vi "readTelemetryDynamicData.vi"(8 "error in (no error)":errorcluster, 10 "Parser":refnum<class "U8ArrayParserAutoIndexing.lvclass">, 11 "M1M3SAL in":refnum<class "M1M3SAL.lvclass">) -> (0 "error out":errorcluster, 2 "EventSummaryState":variant, 3 "M1M3SAL out":refnum<class "M1M3SAL.lvclass">)   [LabVIEW 2016, in "M1M3SupportCommunicator.lvlib" / "M1M3SAL.lvclass"]
uses:
  M1M3SAL.lvclass
  Common_RT_Utilities/U8ArrayParserAutoIndexing/U8ArrayParserAutoIndexing.lvclass
  DataTypes/Topics/TelemetryDynamicData.ctl
  DataTypes/Topics/Parts/Timestamp.ctl
  DataTypes/Topics/M1M3SupportTopics.lvlib
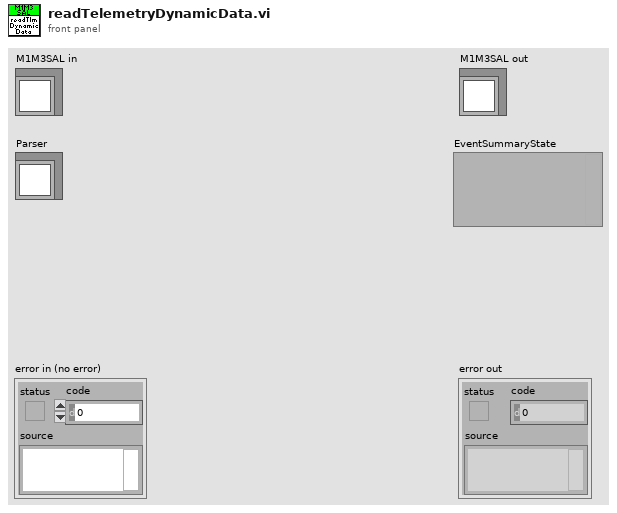
[diagram p1: front panel]
types:
  T1 = typedef "M1M3SupportTopics.lvlib/TelemetryDynamicData.ctl" = cluster{"Timestamp":T2, "AzimuthVelocity":dbl, "ElevationVelocity":dbl, "AzimuthAcceleration":dbl, "ElevationAcceleration":dbl}
  T2 = typedef "M1M3SupportTopics.lvlib/Timestamp.ctl" = dbl
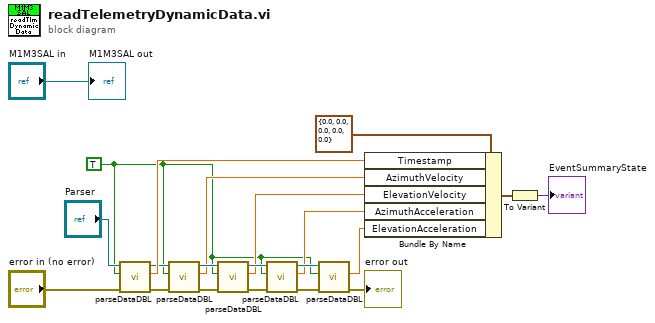
[diagram p0: block diagram]
diagram:
  w1 = TRUE ("OverrideSwapBytes")
  n1 = call "parseDataDBL.vi"("error in (no error)"="error in (no error)", "OverrideSwapBytes"=w1, "U8ArrayParserAutoIndexing in"="Parser") -> ("error out"=w9:errorcluster, "Data"=w16:dbl, "U8ArrayParserAutoIndexing out"=w11:refnum<class "U8ArrayParserAutoIndexing.lvclass">)  [unwired: 6 in]
  n2 = call "parseDataDBL.vi"("error in (no error)"=w9, "OverrideSwapBytes"=w1, "U8ArrayParserAutoIndexing in"=w11) -> ("error out"=w8:errorcluster, "Data"=w7:dbl, "U8ArrayParserAutoIndexing out"=w10:refnum<class "U8ArrayParserAutoIndexing.lvclass">)  [unwired: 6 in]
  n3 = call "parseDataDBL.vi"("error in (no error)"=w8, "OverrideSwapBytes"=w1, "U8ArrayParserAutoIndexing in"=w10) -> ("error out"=w15:errorcluster, "Data"=w6:dbl, "U8ArrayParserAutoIndexing out"=w14:refnum<class "U8ArrayParserAutoIndexing.lvclass">)  [unwired: 6 in]
  n4 = call "parseDataDBL.vi"("error in (no error)"=w15, "OverrideSwapBytes"=w1, "U8ArrayParserAutoIndexing in"=w14) -> ("error out"=w13:errorcluster, "Data"=w5:dbl, "U8ArrayParserAutoIndexing out"=w12:refnum<class "U8ArrayParserAutoIndexing.lvclass">)  [unwired: 6 in]
  n5 = call "parseDataDBL.vi"("error in (no error)"=w13, "OverrideSwapBytes"=w1, "U8ArrayParserAutoIndexing in"=w12) -> ("error out"=→"error out":errorcluster, "Data"=w4:dbl)  [unwired: 6 in, 1 out]
  n6 = Bundle By Name(cluster=T1 {"Timestamp"=0.0, "AzimuthVelocity"=0.0, "ElevationVelocity"=0.0, "AzimuthAcceleration"=0.0, "ElevationAcceleration"=0.0} ("TelemetryDynamicData"), "Timestamp"=w16, "AzimuthVelocity"=w7, "ElevationVelocity"=w6, "AzimuthAcceleration"=w5, "ElevationAcceleration"=w4) -> (w20:T1)
  n7 = To Variant(anything=w20) -> (Variant=→"EventSummaryState":variant)
  "M1M3SAL out" <- "M1M3SAL in"
